vi "init_DAQ_cluster.vi"(9 "Sample rate":dbl=100000.0, 10 "Slow/Zelux frame frequency":dbl=20.0, 11 "Fast/Kinetix frame frequency":dbl=100.0) -> (0 "error out":errorcluster, 3 "tasks cluster":T1)   [LabVIEW 2025]
uses:
  DAQ_tasks_control.ctl
  <vilib>/DAQmx/create/channels.llb/DAQmx Create Channel (AO-Voltage-Basic).vi
  <vilib>/DAQmx/create/channels.llb/DAQmx Create Channel (CO-Pulse Generation-Frequency).vi
  <vilib>/DAQmx/create/channels.llb/DAQmx Create Channel (AI-Voltage-Basic).vi
  <vilib>/DAQmx/configure/timing.llb/DAQmx Timing (Implicit).vi
  <vilib>/DAQmx/configure/timing.llb/DAQmx Timing (Sample Clock).vi
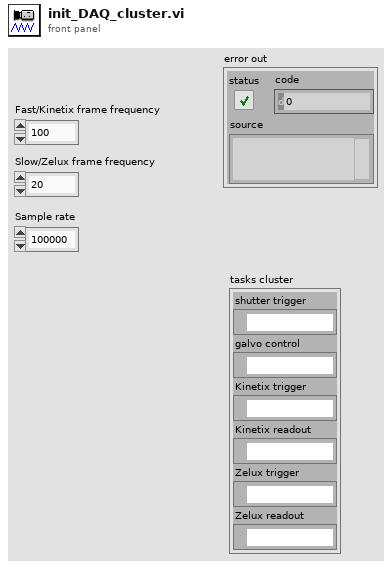
[diagram p1: front panel]
types:
  T1 = cluster{"shutter trigger":refnum<k21>, "galvo control":refnum<k21>, "Kinetix trigger":refnum<k21>, "Kinetix readout":refnum<k21>, "Zelux trigger":refnum<k21>, "Zelux readout":refnum<k21>}
  T2 = typedef "DAQ_tasks_control.ctl" = cluster{"shutter trigger":refnum<k21>, "galvo control":refnum<k21>, "Kinetix trigger":refnum<k21>, "Kinetix readout":refnum<k21>, "Zelux trigger":refnum<k21>, "Zelux readout":refnum<k21>}
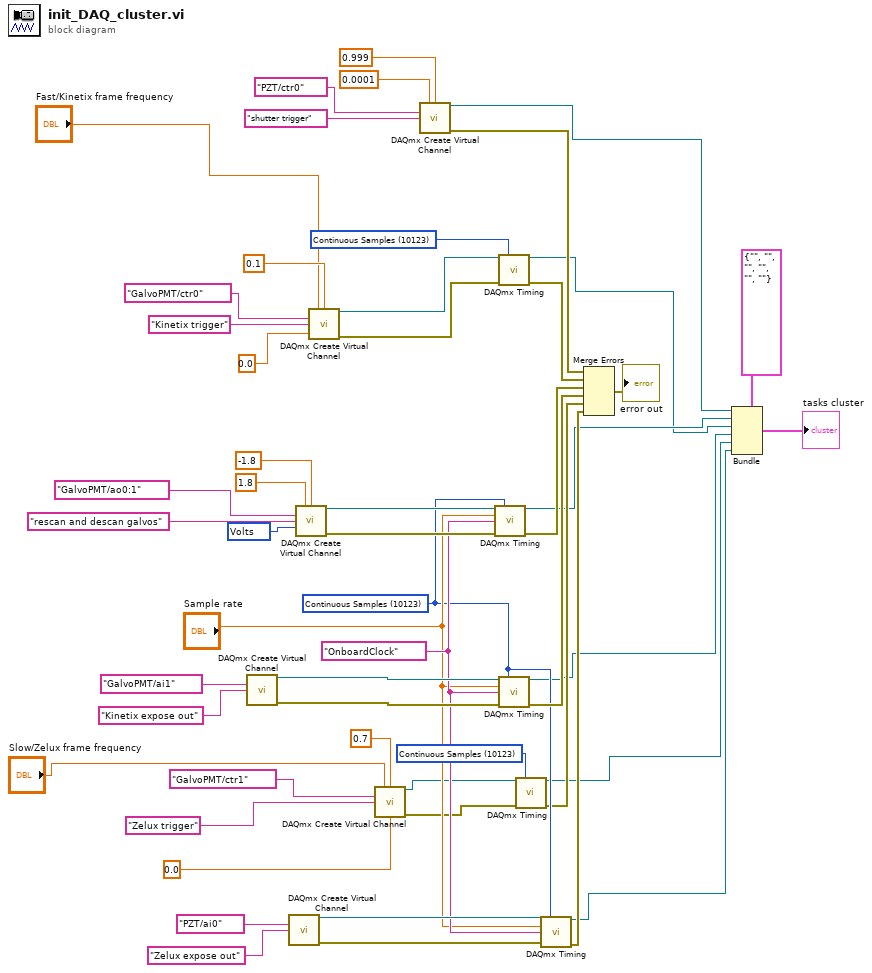
[diagram p0: block diagram]
diagram:
  w12 = 10123 items=["Finite Samples"=10178, "Continuous Samples"=10123, "Hardware Timed Single Point"=12522] ("sample mode")
  w29 = 10123 items=["Finite Samples"=10178, "Continuous Samples"=10123, "Hardware Timed Single Point"=12522] ("sample mode")
  w19 = tag "OnboardClock" ("source")
  w17 = 10123 items=["Finite Samples"=10178, "Continuous Samples"=10123, "Hardware Timed Single Point"=12522] ("sample mode")
  w53 = 10348 items=["Volts"=10348, "From Custom Scale"=10065] ("units")
  n1 = call-poly <vilib>:"DAQmx Create Virtual Channel.vi"("physical channels"=tag "GalvoPMT/ai1", "name to assign"="Kinetix expose out") -> ("task out"=w36:refnum<k21>, "error out"=w37:errorcluster)  [unwired: 12 in]
  n2 = call-poly <vilib>:"DAQmx Create Virtual Channel.vi"("physical channels"=tag "PZT/ai0", "name to assign"="Zelux expose out") -> ("task out"=w20:refnum<k21>, "error out"=w16:errorcluster)  [unwired: 12 in]
  n3 = call-poly <vilib>:"DAQmx Create Virtual Channel.vi"("maximum value"=1.8, "minimum value"=-1.8, "physical channels"=tag "GalvoPMT/ao0:1", "name to assign"="rescan and descan galvos", "units"=w53) -> ("task out"=w41:refnum<k21>, "error out"=w40:errorcluster)  [unwired: 9 in]
  n4 = call-poly <vilib>:"DAQmx Create Virtual Channel.vi"("frequency"="Fast/Kinetix frame frequency", "duty cycle"=0.1, "counter"=tag "GalvoPMT/ctr0", "name to assign"="Kinetix trigger", "initial delay"=0.0) -> ("task out"=w27:refnum<k21>, "error out"=w30:errorcluster)  [unwired: 9 in]
  n5 = call-poly <vilib>:"DAQmx Create Virtual Channel.vi"("frequency"="Slow/Zelux frame frequency", "duty cycle"=0.7, "counter"=tag "GalvoPMT/ctr1", "name to assign"="Zelux trigger", "initial delay"=0.0) -> ("task out"=w11:refnum<k21>, "error out"=w9:errorcluster)  [unwired: 9 in]
  n6 = call-poly <vilib>:"DAQmx Create Virtual Channel.vi"("frequency"=0.0001, "duty cycle"=0.999, "counter"=tag "PZT/ctr0", "name to assign"="shutter trigger") -> ("task out"=w8:refnum<k21>, "error out"=w35:errorcluster)  [unwired: 10 in]
  n7 = call-poly <vilib>:"DAQmx Timing.vi"("task/channels in"=w41, "sample mode"=w17, "rate"="Sample rate", "source"=w19, "error in"=w40) -> ("task out"=w2:refnum<k21>, "error out"=w33:errorcluster)  [unwired: 9 in]
  n8 = call-poly <vilib>:"DAQmx Timing.vi"("task/channels in"=w27, "sample mode"=w29, "error in"=w30) -> ("task out"=w1:refnum<k21>, "error out"=w28:errorcluster)  [unwired: 11 in]
  n9 = call-poly <vilib>:"DAQmx Timing.vi"("task/channels in"=w36, "sample mode"=w17, "rate"="Sample rate", "source"=w19, "error in"=w37) -> ("task out"=w7:refnum<k21>, "error out"=w32:errorcluster)  [unwired: 9 in]
  n10 = call-poly <vilib>:"DAQmx Timing.vi"("task/channels in"=w11, "sample mode"=w12, "error in"=w9) -> ("task out"=w6:refnum<k21>, "error out"=w10:errorcluster)  [unwired: 11 in]
  n11 = call-poly <vilib>:"DAQmx Timing.vi"("task/channels in"=w20, "sample mode"=w17, "rate"="Sample rate", "source"=w19, "error in"=w16) -> ("task out"=w5:refnum<k21>, "error out"=w15:errorcluster)  [unwired: 9 in]
  n12 = Merge Errors(w35, w28, w33, w32, w10, w15) -> (→"error out":errorcluster)
  n13 = Bundle(cluster=T2 {"shutter trigger"="", "galvo control"="", "Kinetix trigger"="", "Kinetix readout"="", "Zelux trigger"="", "Zelux readout"=""}, "shutter trigger"=w8, "galvo control"=w2, "Kinetix trigger"=w1, "Kinetix readout"=w7, "Zelux trigger"=w6, "Zelux readout"=w5) -> (→"tasks cluster":T2)
